vi "LEIN to Canbus frame.vi"(7 "CMD":T2={"SID"=0, "ANF"=FALSE, "CMD"=enum."TASK", "DATA"=[]}, 11 "error in (no error)":errorcluster) -> (3 "Data Length":u32, 6 "Data":u8[](array[numeric]), 8 "Complete frame":T1 {"Data" format="%.0x"; "ArbitrationId" format="%.0x"; "Timestamp" format="%<%I:%M:%S%3u %p\n%m/%d/%Y>T"}, 10 "Is remote":u8, 14 "ArbitrationID":u32, 15 "error out":errorcluster)   [LabVIEW 2011]
uses:
  Defenitions/LEIN CMD Cluster.ctl
  Defenitions/LEIN CMD List.ctl
  <vilib>/nican/nican.llb/CanFrameTimed.ctl
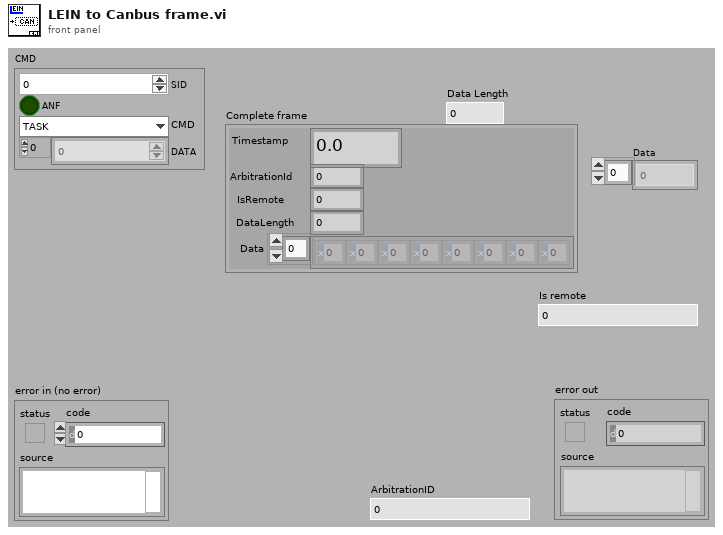
[diagram p1: front panel]
types:
  T1 = typedef "CanFrameTimed.ctl" = cluster{"Timestamp":dbl, "ArbitrationId":u32, "IsRemote":u8, "DataLength":u8, "Data":u8[]}
  T2 = typedef "LEIN CMD Cluster.ctl" = cluster{"SID":u8, "ANF":bool, "CMD":T3, "DATA":u8[]}
  T3 = typedef "LEIN CMD List.ctl" = enum8{"ACTI", "TASK", "RES0", "STAT", "RES1", "RES2", "RES3", "USER"}
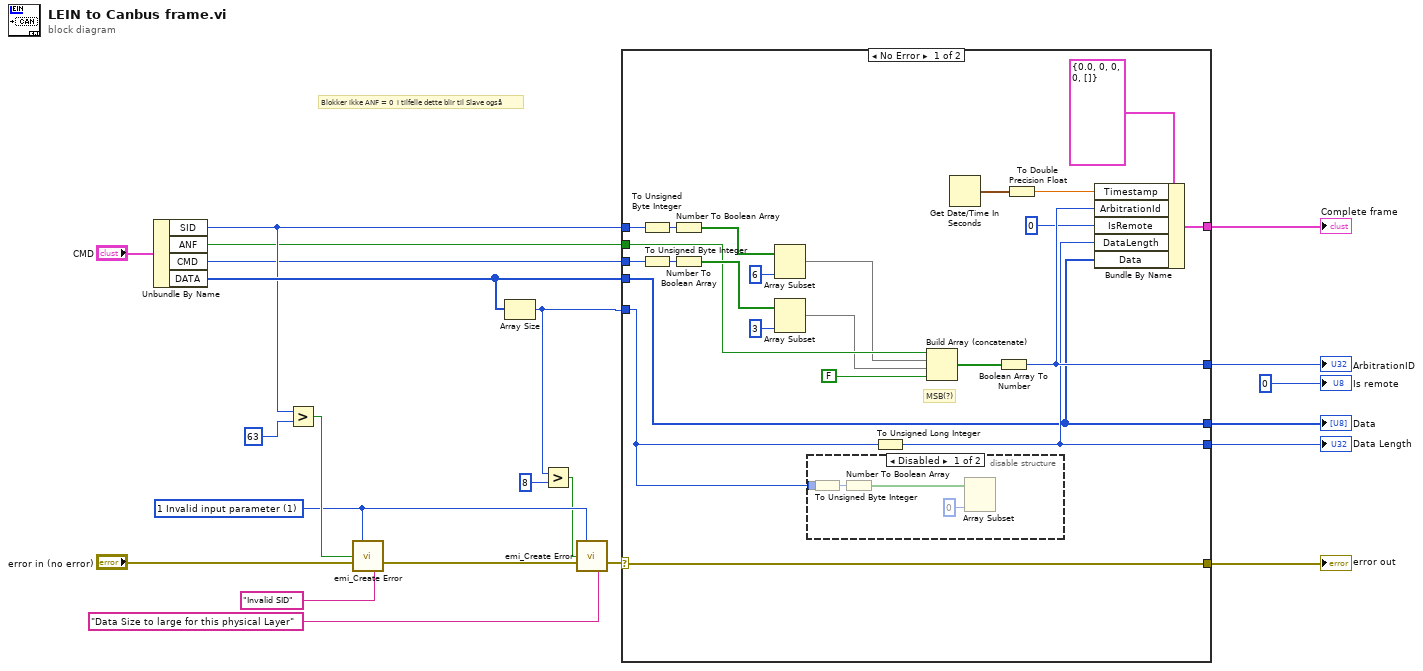
[diagram p0: block diagram]
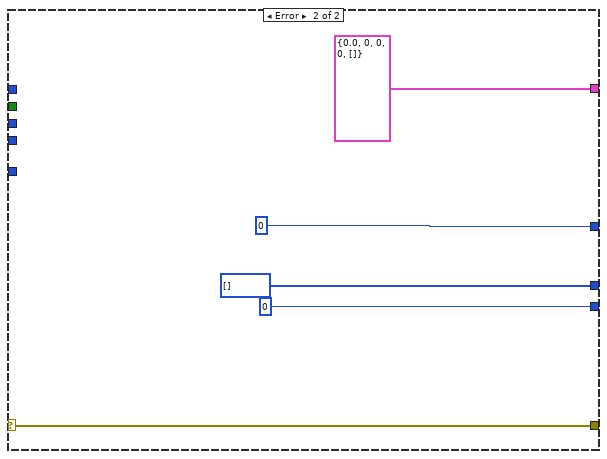
[diagram p3: hidden frame]
diagram:
  w12 = 1 items=["0 No Error"=0, "1 Invalid input parameter"=1, "6 Generic file IO "=6, "7 File not Found"=7, "35 Generic Pring Error"=35, "37 Device not Found"=37, "39 Device Unit Error"=39, "40 Could fot Open Device"=40, "42 Generic Error"=42, "52 Unknown Message"=52, "98 Bad File type"=98, "99 Bad File Version"=99, "100 Bad Data in File"=100, "1018 Unspecefied Error"=1018, "1041 Incorrect Password"=1041, "1043 Feature not in this version"=1043, "1109 Unsuported Data type"=1109, "1444 Did not close sucessfully"=1444] ("Error Code")
  # "Blokker ikke ANF = 0  i tilfelle dette blir til Slave også"
  n1 = Unbundle By Name("CMD") -> ("SID"=w3:u8, "ANF"=w2:bool, "CMD"=w1:T3, "DATA"=w5:u8[])
  n2 = Greater?(x=w3, y=u8 63) -> (0:w15:bool)
  n3 = call "emi_Create Error.vi"("Error Code"=w12, "Error(T)"=w15, "error in (no error)"="error in (no error)", "Append String(\"\")"="Invalid SID" ("Append String(\"\")")) -> ("error out"=w13:errorcluster)  [unwired: 11 in]
  n4 = Array Size(array=w5) -> (size(s)=w6:i32)
  n5 = Greater?(x=w6, y=8) -> (0:w11:bool)
  n6 = call "emi_Create Error.vi"("Error Code"=w12, "Error(T)"=w11, "error in (no error)"=w13, "Append String(\"\")"="Data Size to large for this physical Layer" ("Append String(\"\")")) -> ("error out"=w8:errorcluster)  [unwired: 11 in]
  n7 = case shown="No Error" w8 {
    selector: w8 -> [w34 w54]
    tunnel: [w27 u32 0] -> w22
    tunnel: w2 -> [w39 _]
    tunnel: w1 -> [w36 _]
    tunnel: w3 -> [w35 _]
    tunnel: w6 -> [w33 _]
    tunnel: [w34 w54] -> w21
    tunnel: [w25 u32 0] -> w20
    tunnel: w5 -> [w24 _]
    tunnel: [w24 u8[] [] ("DATA")] -> w18
    tunnel: [w30 T1 {"Timestamp"=0.0, "ArbitrationId"=0, "IsRemote"=0, "DataLength"=0, "Data"=[]} ("CAN FRAME TIMED")] -> w17
    frame No Error {
      # "MSB(?)"
      n8 = To Unsigned Byte Integer(number=w35) -> (unsigned 8bit integer=w44:u8)
      n9 = To Unsigned Byte Integer(number=w36) -> (unsigned 8bit integer=w45:u8)
      n10 = Number To Boolean Array(number=w44) -> (Boolean array=w42:bool[])
      n11 = Number To Boolean Array(number=w45) -> (Boolean array=w43:bool[])
      n12 = Array Subset(array=w42, length=6) -> (w37:bool[])  [unwired: 1 in]
      n13 = Array Subset(array=w43, length=3) -> (w38:bool[])  [unwired: 1 in]
      n14 = disable-structure shown="Disabled" {
        disable-tunnel: w33 -> [w49 _]
        frame Disabled {
          n15 = To Unsigned Byte Integer(number=w49) -> (unsigned 8bit integer=w48:u8)
          n16 = Number To Boolean Array(number=w48) -> (Boolean array=w47:bool[])
          n17 = Array Subset(array=w47, length=0) -> ()  [unwired: 1 in, 1 out]
        }
        frame Enabled {
        }
      }
      n18 = To Unsigned Long Integer(number=w33) -> (unsigned 32bit integer=w25:u32)
      n19 = Build Array (concatenate)(w39, w37, w38, FALSE ("ANF")) -> (w32:bool[])
      n20 = Get Date/Time In Seconds() -> (seconds since 1Jan1904=w29:timestamp)
      n21 = Boolean Array To Number(Boolean array=w32) -> (number=w27:u32)
      n22 = To Double Precision Float(number=w29) -> (double precision float=w28:dbl)
      n23 = Bundle By Name(cluster=T1 {"Timestamp"=0.0, "ArbitrationId"=0, "IsRemote"=0, "DataLength"=0, "Data"=[]} ("CAN FRAME TIMED"), "Timestamp"=w28, "ArbitrationId"=w27, "IsRemote"=u8 0, "DataLength"=w25, "Data"=w24) -> (w30:T1)
    }
    frame Error {
    }
  }
  "ArbitrationID" <- w22
  "Data Length" <- w20
  "error out" <- w21
  "Data" <- w18
  "Complete frame" <- w17
  "Is remote" <- u8 0 ("Arb ID 2")
